vi "7.7.4-Forebrain_to_OCU-UDPClient.vi"() -> ()   [LabVIEW 2010]
doc: "This VI implements a client for the Named Service UDP Server.vi.\nIt connects to a service by specifying the server address and the name of the service. After sending a 'Hello' string to the server, the client receives the string sent by the server, displays the string and closes the connection.\n\n<b>Note:</b> This VI is built to work with the Named Service UDP Server.vi in UDP.llb."
uses:
  6-OCU Neurons/CommonIndicators.ctl
  4-High Neurons/4.4-How Sensor Typedef.ctl
  7.0-Global.vi
panel:
  out "Main Indicators":T1
  out "String":string
  out "error out":errorcluster
  in  "error in":errorcluster
  # "Instructions:\n1. Open Named Service UDP Server.vi located in the same library.\n2. Follow the instructions on it's front panel.\n\nNote: This VI is built to work with the Named Service UDP Server.vi in UDP.llb."
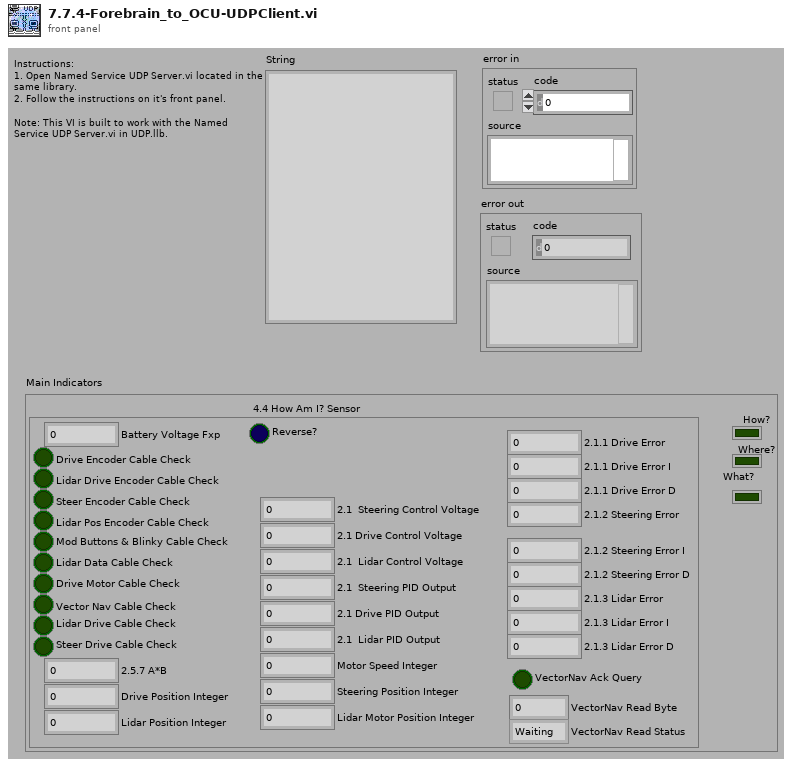
[diagram p1: front panel]
types:
  T1 = typedef "CommonIndicators.ctl" = cluster{"4.4 How Am I? Sensor":T2, "How?":bool, "Where?":bool, "What?":bool}
  T2 = typedef "4.4-How Sensor Typedef.ctl" = cluster{"Motor Speed Integer":i32, "Drive Position Integer":i32, "Lidar Position Integer":i32, "Lidar Motor Position Integer":i32, "Steering Position Integer":i32, "Battery Voltage Fxp":dbl, "Drive Encoder Cable Check":bool, "Lidar Drive Encoder Cable Check":bool, "Steer Encoder Cable Check":bool, "Lidar Pos Encoder Cable Check":bool, "Mod Buttons & Blinky Cable Check":bool, "Lidar Data Cable Check":bool, "Drive Motor Cable Check":bool, "Vector Nav Cable Check":bool, "Lidar Drive Cable Check":bool, "Steer Drive Cable Check":bool, "Reverse?":bool, "2.1  Steering Control Voltage":dbl, "2.1 Drive Control Voltage":dbl, "2.1  Lidar Control Voltage":dbl, "2.5.7 A*B":dbl, "2.1  Steering PID Output":dbl, "2.1 Drive PID Output":dbl, "2.1  Lidar PID Output":dbl, "2.1.1 Drive Error":dbl, "2.1.1 Drive Error I":dbl, "2.1.1 Drive Error D":dbl, "2.1.2 Steering Error":dbl, "2.1.2 Steering Error I":dbl, "2.1.2 Steering Error D":dbl, "2.1.3 Lidar Error":dbl, "2.1.3 Lidar Error I":dbl, "2.1.3 Lidar Error D":dbl, "VectorNav Ack Query":bool, "VectorNav Read Byte":u8, "VectorNav Read Status":enum16{"Waiting", "Reading", "Done"}}
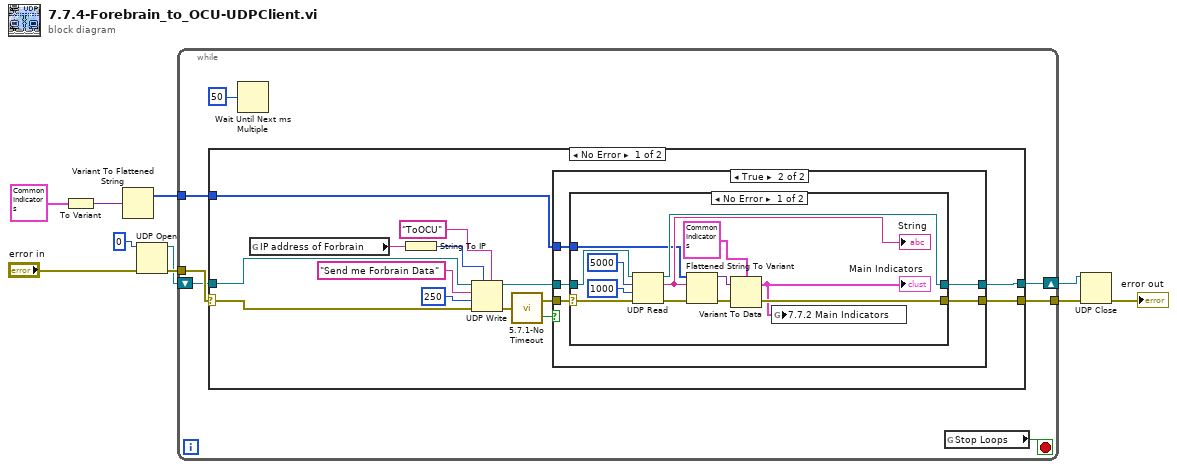
[diagram p0: block diagram]
diagram:
  n1 = To Variant(anything=T1 {"4.4 How Am I? Sensor"={"Motor Speed Integer"=0, "Drive Position Integer"=0, "Lidar Position Integer"=0, "Lidar Motor Position Integer"=0, "Steering Position Integer"=0, "Battery Voltage Fxp"=0.0, "Drive Encoder Cable Check"=FALSE, "Lidar Drive Encoder Cable Check"=FALSE, "Steer Encoder Cable Check"=FALSE, "Lidar Pos Encoder Cable Check"=FALSE, "Mod Buttons & Blinky Cable Check"=FALSE, "Lidar Data Cable Check"=FALSE, "Drive Motor Cable Check"=FALSE, "Vector Nav Cable Check"=FALSE, "Lidar Drive Cable Check"=FALSE, "Steer Drive Cable Check"=FALSE, "Reverse?"=FALSE, "2.1  Steering Control Voltage"=0.0, "2.1 Drive Control Voltage"=0.0, "2.1  Lidar Control Voltage"=0.0, "2.5.7 A*B"=0.0, "2.1  Steering PID Output"=0.0, "2.1 Drive PID Output"=0.0, "2.1  Lidar PID Output"=0.0, "2.1.1 Drive Error"=0.0, "2.1.1 Drive Error I"=0.0, "2.1.1 Drive Error D"=0.0, "2.1.2 Steering Error"=0.0, "2.1.2 Steering Error I"=0.0, "2.1.2 Steering Error D"=0.0, "2.1.3 Lidar Error"=0.0, "2.1.3 Lidar Error I"=0.0, "2.1.3 Lidar Error D"=0.0, "VectorNav Ack Query"=FALSE, "VectorNav Read Byte"=0, "VectorNav Read Status"=enum."Waiting"}, "How?"=FALSE, "Where?"=FALSE, "What?"=FALSE} ("data")) -> (Variant=w3:variant)
  n2 = Variant To Flattened String(Variant=w3) -> (1:w2:i16[])  [unwired: 1 out]
  n3 = UDP Open(8:"error in", 11:u16 0) -> (port=w7:refnum<k16>, 0:w8:errorcluster)  [unwired: 3 in, 1 out]
  n4 = while {
    tunnel: [w17] -> w5
    tunnel: w8 -> [w16]
    shift-right: [w14] -> w6
    shift-left: w7 -> [w15]
    tunnel: w2 -> [w12]
    stop <- w11 stop-if-true
    n5 = case shown="No Error" w16 {
      selector: w16 -> [w31 w55]
      tunnel: [w26 w55] -> w17
      tunnel: w15 -> [w30 w54]
      tunnel: [w25 w54] -> w14
      tunnel: w12 -> [w20 _]
      frame No Error {
        n6 = global read "7.0-Global.vi" "IP address of Forbrain"() -> (w19:string)
        n7 = String To IP(1:w19) -> (0:w29:u32)
        n8 = UDP Write(address=w29, port or service name="ToOCU", connection ID=w30, data in="Send me Forbrain Data", 8:w31, 9:250 ("timeout ms (25000)")) -> (error out=w24:errorcluster, 3:w27:refnum<k16>)
        n9 = call "5.7.1-No Timeout.vi"("error in (no error)"=w24) -> ("No Timeout"=w22:bool, "error out"=w23:errorcluster)
        n10 = case shown="True" w22 {
          tunnel: w23 -> [w33 w38]
          tunnel: w27 -> [w32 w37]
          tunnel: [w32 w36] -> w25
          tunnel: [w33 w35] -> w26
          tunnel: w20 -> [_ w34]
          frame False {
          }
          frame True {
            n11 = case shown="No Error" w38 {
              selector: w38 -> [w51 w52]
              tunnel: w37 -> [w50 w53]
              tunnel: [w48 w53] -> w36
              tunnel: [w41 w52] -> w35
              tunnel: w34 -> [w45 _]
              frame No Error {
                n12 = UDP Read(connection ID=w50, max size (548)=5000, timeout ms (25000)=1000, 8:w51) -> (data out=w46:string, error out=w42:errorcluster, 3:w48:refnum<k16>)  [unwired: 2 out]
                "String" <- w46
                n13 = Flattened String To Variant(4:w42, 6:w46, 7:w45) -> (0:w43:errorcluster, 3:w44:variant)
                n14 = Variant To Data(error in=w43, Variant=w44, type=T1 {"4.4 How Am I? Sensor"={"Motor Speed Integer"=0, "Drive Position Integer"=0, "Lidar Position Integer"=0, "Lidar Motor Position Integer"=0, "Steering Position Integer"=0, "Battery Voltage Fxp"=0.0, "Drive Encoder Cable Check"=FALSE, "Lidar Drive Encoder Cable Check"=FALSE, "Steer Encoder Cable Check"=FALSE, "Lidar Pos Encoder Cable Check"=FALSE, "Mod Buttons & Blinky Cable Check"=FALSE, "Lidar Data Cable Check"=FALSE, "Drive Motor Cable Check"=FALSE, "Vector Nav Cable Check"=FALSE, "Lidar Drive Cable Check"=FALSE, "Steer Drive Cable Check"=FALSE, "Reverse?"=FALSE, "2.1  Steering Control Voltage"=0.0, "2.1 Drive Control Voltage"=0.0, "2.1  Lidar Control Voltage"=0.0, "2.5.7 A*B"=0.0, "2.1  Steering PID Output"=0.0, "2.1 Drive PID Output"=0.0, "2.1  Lidar PID Output"=0.0, "2.1.1 Drive Error"=0.0, "2.1.1 Drive Error I"=0.0, "2.1.1 Drive Error D"=0.0, "2.1.2 Steering Error"=0.0, "2.1.2 Steering Error I"=0.0, "2.1.2 Steering Error D"=0.0, "2.1.3 Lidar Error"=0.0, "2.1.3 Lidar Error I"=0.0, "2.1.3 Lidar Error D"=0.0, "VectorNav Ack Query"=FALSE, "VectorNav Read Byte"=0, "VectorNav Read Status"=enum."Waiting"}, "How?"=FALSE, "Where?"=FALSE, "What?"=FALSE} ("data")) -> (error out=w41:errorcluster, data=w40:T1)
                "Main Indicators" <- w40
                n15 = global write "7.0-Global.vi" "7.7.2 Main Indicators"(w40) -> ()
              }
              frame Error {
              }
            }
          }
        }
      }
      frame Error {
      }
    }
    n16 = Wait Until Next ms Multiple(millisecond multiple=u32 50) -> ()  [unwired: 1 out]
    n17 = global read "7.0-Global.vi" "Stop Loops"() -> (w11:bool)
  }
  n18 = UDP Close(connection ID=w6, 8:w5) -> (error out=→"error out":errorcluster)  [unwired: 1 out]
